vi "e-l_gate.vi"(8 "error in (no error)":errorcluster, 10 "input complex waveform":cluster{"t0":dbl, "dt":dbl, "Y":cdb[]}={"t0"=0.0, "dt"=1.0, "Y"=[]} {"Y" format="%.3f"; "dt" format="%^.2e"; "t0" format="%.4f"}, 11 "Modulation Parameters In":T1={"RX Parameters"={"RX Oversample Factor"=4, "RX Sample Rate"=4000000.0, "Synchronization Options"={"Synchronization Method"=enum."Fixed Offset", "Symbol Timing Recovery Method "=enum."MT Allign To Ideal Symbols", "Fixed Offset"=0.0, "Frame Detection Method"=enum."", "Correct Frequency Offset"=FALSE}, "Channel Estimation/Equalization Parameters"={"Equalization Method"=enum."", "Channel Estimate Length"=0.0, "Equalizer Length"=0.0, "Equalizer Delay"=0.0}}, "TX/RX Shared Parameters"={"Modulation Type"=enum."OOK", "Packet Length"=128, "# of Iterations"=0.0, "Pulse Shaping Parameters"={"Pulse Shaping Filter"=enum."none", "Filter Length (symbols)"=32, "Filter Parameter"=0.8, "modulation type"=enum."FSK"}, "Header/Tail Control Information"={"Training Sequence Type"=enum."", "Zero Pad Length"=0.0}}}) -> (0 "error out":errorcluster, 1 "alignment offset (samples)":i32, 2 "aligned complex waveform":cluster{"t0":dbl, "dt":dbl, "Y":cdb[]} {"Y" format="%.3f"; "dt" format="%^.2e"; "t0" format="%.4f"}, 3 "Modulation Parameters Out":T1={"RX Parameters"={"RX Oversample Factor"=4, "RX Sample Rate"=4000000.0, "Synchronization Options"={"Synchronization Method"=enum."Fixed Offset", "Symbol Timing Recovery Method "=enum."MT Allign To Ideal Symbols", "Fixed Offset"=0.0, "Frame Detection Method"=enum."", "Correct Frequency Offset"=FALSE}, "Channel Estimation/Equalization Parameters"={"Equalization Method"=enum."", "Channel Estimate Length"=0.0, "Equalizer Length"=0.0, "Equalizer Delay"=0.0}}, "TX/RX Shared Parameters"={"Modulation Type"=enum."OOK", "Packet Length"=128, "# of Iterations"=0.0, "Pulse Shaping Parameters"={"Pulse Shaping Filter"=enum."none", "Filter Length (symbols)"=32, "Filter Parameter"=0.8, "modulation type"=enum."FSK"}, "Header/Tail Control Information"={"Training Sequence Type"=enum."", "Zero Pad Length"=0.0}}})   [LabVIEW 2012]
uses:
  <vilib>/Analysis/2dsp.llb/Decimate (single shot, CDB).vi
  <vilib>/Analysis/NI_AALPro.lvlib
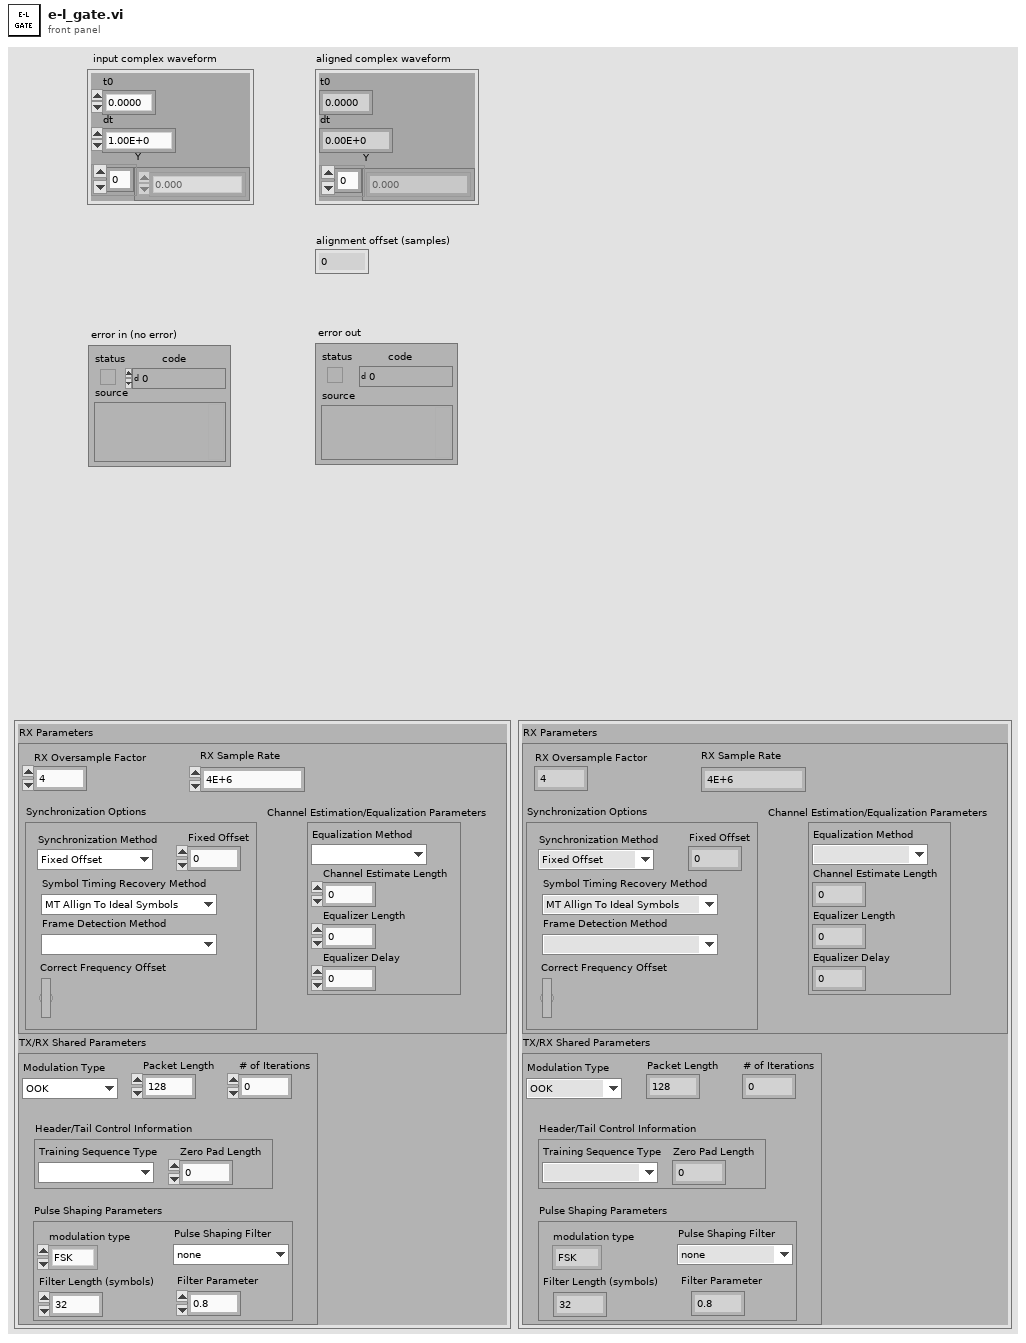
[diagram p1: front panel]
types:
  T1 = cluster{"RX Parameters":cluster{"RX Oversample Factor":i32, "RX Sample Rate":dbl, "Synchronization Options":cluster{"Synchronization Method":enum16{"Fixed Offset", "Timing Estimation", "Joint Timing and Channel Estimation"}, "Symbol Timing Recovery Method ":enum16{"MT Allign To Ideal Symbols", "Maximum Energy", "Early-Late Gate", "Gardner", "Fixed Offset"}, "Fixed Offset":dbl, "Frame Detection Method":enum16{""}, "Correct Frequency Offset":bool}, "Channel Estimation/Equalization Parameters":cluster{"Equalization Method":enum16{""}, "Channel Estimate Length":dbl, "Equalizer Length":dbl, "Equalizer Delay":dbl}}, "TX/RX Shared Parameters":cluster{"Modulation Type":enum16{"OOK", "FSK"}, "Packet Length":i32, "# of Iterations":dbl, "Pulse Shaping Parameters":cluster{"Pulse Shaping Filter":enum16{"none", "Raised Cosine", "Root Raised Cos", "Gaussian"}, "Filter Length (symbols)":i32, "Filter Parameter":dbl, "modulation type":enum16{"FSK", "PSK", "QAM", "MSK", "PAM", "ASK", "CPM"}}, "Header/Tail Control Information":cluster{"Training Sequence Type":enum16{""}, "Zero Pad Length":dbl}}}
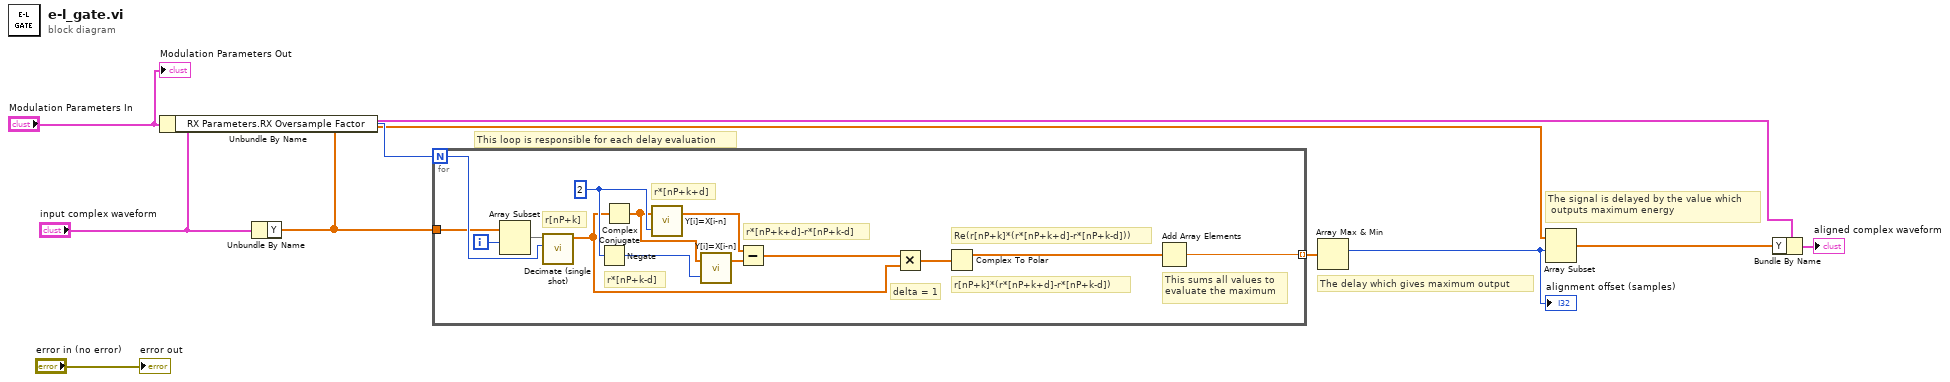
[diagram p0: block diagram]
diagram:
  # "The signal is delayed by the value which\n outputs maximum energy"
  # "The delay which gives maximum output"
  # "This loop is responsible for each delay evaluation"
  n1 = Unbundle By Name("Modulation Parameters In") -> ("RX Parameters.RX Oversample Factor"=w9:i32)
  n2 = Unbundle By Name("input complex waveform") -> ("Y"=w3:cdb[])
  n3 = for {
    N: w9 -> [w12]
    tunnel: [w16] -> w7 mode=indexing
    tunnel: w3 -> [w11]
    i -> [w10]
    w22 = 2 ("shifts: n")
    # "delta = 1"
    # "This sums all values to\nevaluate the maximum"
    # "Re(r[nP+k]*(r*[nP+k+d]-r*[nP+k-d]))"
    # "r[nP+k]*(r*[nP+k+d]-r*[nP+k-d])"
    # "r*[nP+k+d]-r*[nP+k-d]"
    # "r*[nP+k-d]"
    # "r*[nP+k+d]"
    # "r[nP+k]"
    n4 = Array Subset(array=w11, index=w10) -> (w13:cdb[])  [unwired: 1 in]
    n5 = call-poly <vilib>:"Decimate (single shot).vi"("decimating factor"=w12, "X"=w13) -> ("Decimated Array"=w14:cdb[])  [unwired: 8 in, 1 out]
    n6 = Negate(x=w22) -> (-x=w23:i32)
    n7 = Complex Conjugate(1:w14) -> (0:w21:cdb[])
    n8 = call <vilib>:"Y[i]=X[i-n].vi"("shifts: n"=w22, "Input Array"=w21) -> ("Shifted Array"=w20:dbl[])  [unwired: 1 out]
    n9 = call <vilib>:"Y[i]=X[i-n].vi"("shifts: n"=w23, "Input Array"=w21) -> ("Shifted Array"=w19:dbl[])  [unwired: 1 out]
    n10 = Subtract(x=w20, y=w19) -> (x-y=w18:dbl[])
    n11 = Multiply(x=w18, y=w14) -> (x*y=w17:cdb[])
    n12 = Complex To Polar(r * e^(i*theta)=w17) -> (r=w15:dbl[])  [unwired: 1 out]
    n13 = Add Array Elements(numeric array=w15) -> (sum=w16:dbl)
  }
  n14 = Array Max & Min(array=w7) -> (max index (indices)=w2:i32)  [unwired: 3 out]
  "alignment offset (samples)" <- w2
  n15 = Array Subset(array=w3, index=w2) -> (w5:cdb[])  [unwired: 1 in]
  n16 = Bundle By Name(cluster="input complex waveform", "Y"=w5) -> (→"aligned complex waveform":cluster{"t0":dbl, "dt":dbl, "Y":cdb[]})
  "error out" <- "error in (no error)"
  "Modulation Parameters Out" <- "Modulation Parameters In"
